vi "pb-reset.vi"(8 "error in (no error)":errorcluster, 11 "path in":path=path "C:/SpinCore/SpinAPI/dll/spinapi64.dll") -> (0 "error out":errorcluster, 3 "path out":path)   [LabVIEW 2014]
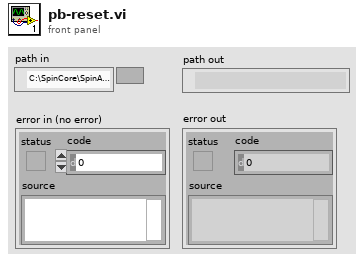
[diagram p1: front panel]
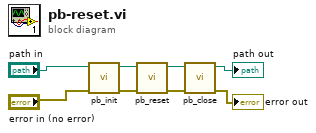
[diagram p0: block diagram]
diagram:
  n1 = call "pb_init.vi"("error in (no error)"="error in (no error)", "path in"="path in") -> ("error out"=w3:errorcluster, "path out"=w4:path)  [unwired: 8 in]
  n2 = call "pb_reset.vi"("error in (no error)"=w3, "path in"=w4) -> ("error out"=w1:errorcluster, "path out"=w2:path)  [unwired: 8 in]
  n3 = call "pb_close.vi"("error in (no error)"=w1, "path in"=w2) -> ("error out"=→"error out":errorcluster, "path out"=→"path out":path)  [unwired: 8 in]
